vi "Untitled 3.vi"() -> ()   [LabVIEW 2020]
panel:
  in  "button":bool
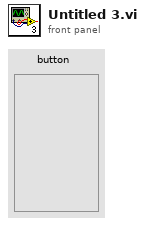
[diagram p1: front panel]
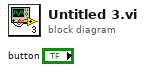
[diagram p0: block diagram]
diagram:
